vi "OSICS_Get_Power_Limit-SWT-APC.vi"(7 "OSICS slot":i32=1 min=1 max=8 step=1, 8 "error in":errorcluster, 11 "VISA IN":refnum<visa-resource-name>) -> (0 "error out":errorcluster, 2 "Power Limit":bool, 3 "VISA OUT":refnum<visa-resource-name>, 5 "ERR":i32)   [LabVIEW 2014, in "OSICS_LIB.lvlib"]
doc: "This Vi reads the power and ENABLED state of the OSICS module SWT-APC in mode Full-Band depending on the input power unit."
uses:
  OSICS_LIB.lvlib
panel:
  # "Basic Function to read the power limit\nof the OSICS SWT APC"
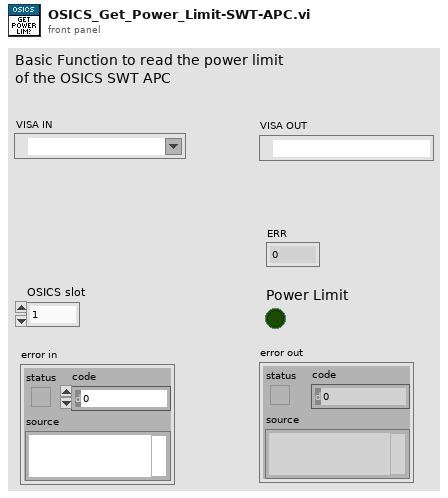
[diagram p1: front panel]
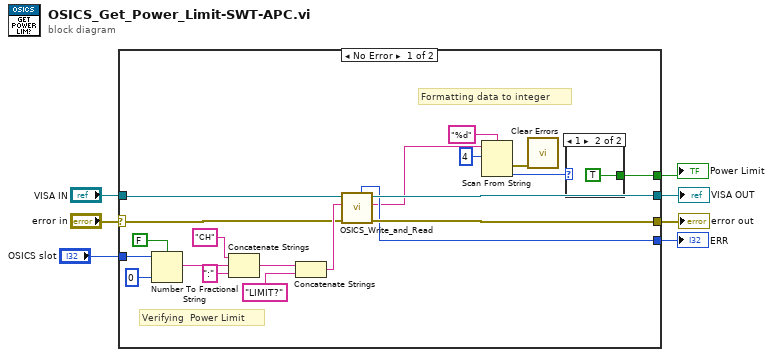
[diagram p0: block diagram]
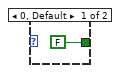
[diagram p2: hidden frame]
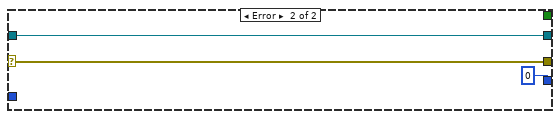
[diagram p3: hidden frame]
diagram:
  n1 = case shown="No Error" "error in" {
    selector: "error in" -> [w15 w31]
    tunnel: "VISA IN" -> [w14 w32]
    tunnel: [w27 w32] -> w6
    tunnel: [w26 w31] -> w5
    tunnel: [w16 0 ("ERR")] -> w3
    tunnel: "OSICS slot" -> [w25 _]
    tunnel: [w13 _] -> w1
    frame No Error {
      # "Formatting data to integer"
      # "Verifying  Power Limit"
      n2 = Number To Fractional String(use system decimal point (T)=FALSE, number=w25, precision (6)=i16 0) -> (F-format string=w21:string)  [unwired: 1 in]
      n3 = Concatenate Strings("CH" ("string"), w21, ":" ("string")) -> (w19:string)
      n4 = Concatenate Strings(w19, "LIMIT?" ("string")) -> (w17:string)
      n5 = call "OSICS_Write_and_Read.vi"("error in (no error)"=w15, "String to Send"=w17, "VISA IN"=w14) -> ("error out"=w26:errorcluster, "Message Available"=w8:string, "VISA OUT"=w27:refnum<visa-resource-name>, "ERR"=w16:i32)  [unwired: 5 in]
      n6 = Scan From String(format string="%d", input string=w8, initial scan location=u32 4) -> (error out=w12:errorcluster, output 1=w10:i32)  [unwired: 2 in, 2 out]
      n7 = call <vilib>:"Clear Errors.vi"("error in (no error)"=w12) -> ()  [unwired: 5 in, 2 out]
      n8 = case shown="1" w10 {
        tunnel: [FALSE TRUE] -> w13
        frame 0, Default {
        }
        frame 1 {
        }
      }
    }
    frame Error {
    }
  }
  "error out" <- w5
  "VISA OUT" <- w6
  "ERR" <- w3
  "Power Limit" <- w1
